vi "TEST_get_SampleHandler_state.vi"() -> ()   [LabVIEW 2017]
uses:
  <vilib>/Instr/_visa.llb/VISA Configure Serial Port (Instr).vi
panel:
  out "文字列":string
  in  "VISAリソース名":refnum<visa-resource-name>
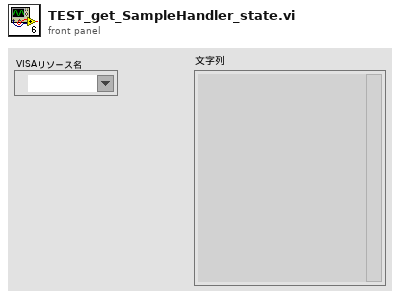
[diagram p1: front panel]
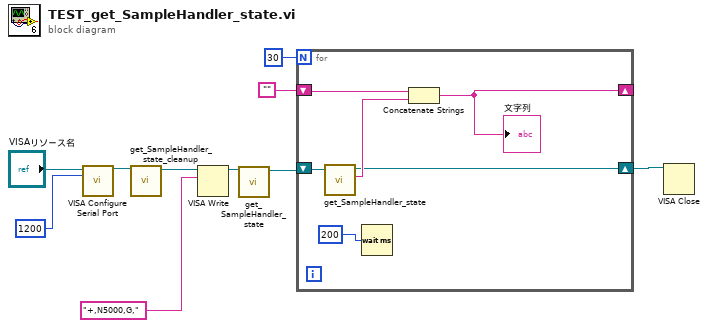
[diagram p0: block diagram]
diagram:
  n1 = call-poly "VISA Configure Serial Port"("VISA resource name"="VISAリソース名", "baud rate (9600)"=1200) -> ("VISA resource name out"=w4:refnum<visa-resource-name>)  [unwired: 12 in, 1 out]
  n2 = call "get_SampleHandler_state_cleanup.vi"("VISAリソース名"=w4) -> ("VISAリソース名（出力）"=w3:refnum<visa-resource-name>)  [unwired: 9 in, 1 out]
  n3 = VISA Write(VISA resource name=w3, write buffer="+,N5000,G,") -> (VISA resource name out=w2:refnum<visa-resource-name>)  [unwired: 1 in, 2 out]
  n4 = call "get_SampleHandler_state.vi"("VISAリソース名"=w2) -> ("VISAリソース名（出力）"=w1:refnum<visa-resource-name>)  [unwired: 8 in, 2 out]
  n5 = for {
    N: 30 -> [_]
    shift-right: [w12] -> _
    shift-left: "" -> [w14]
    shift-right: [w11] -> w5
    shift-left: w1 -> [w15]
    n6 = call "get_SampleHandler_state.vi"("VISAリソース名"=w15) -> ("response"=w13:string, "VISAリソース名（出力）"=w11:refnum<visa-resource-name>)  [unwired: 8 in, 1 out]
    n7 = Wait (ms)(milliseconds to wait=200) -> ()  [unwired: 1 out]
    n8 = Concatenate Strings(w14, w13) -> (w12:string)
    "文字列" <- w12
  }
  n9 = VISA Close(VISA resource name=w5) -> ()  [unwired: 1 in, 1 out]
